vi "Get Index Directory Path.vi"(8 "error in (no error)":errorcluster) -> (0 "error out":errorcluster, 3 "Index Directory":path)   [LabVIEW 2020, in "Paths.lvlib"]
doc: "Generates the default configuration path. \nWhen called from the development environement, the default config path is the /Config relative to the project path.\nWhen called from a built exe the default config path is at C:\\Users\\<username>\\AppData\\Local\\<CompanyName>\\<ProductName> where company name and product name are the ones configured in the build specification.\nOn Linux the default config directory is \\home\\lvuser\\natinst\\bin\\config."
uses:
  Paths.lvlib
  <vilib>/Utility/sysdir.llb/System Directory Type.ctl
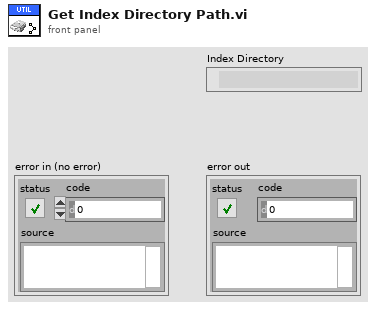
[diagram p1: front panel]
types:
  T1 = typedef "System Directory Type.ctl" = i32
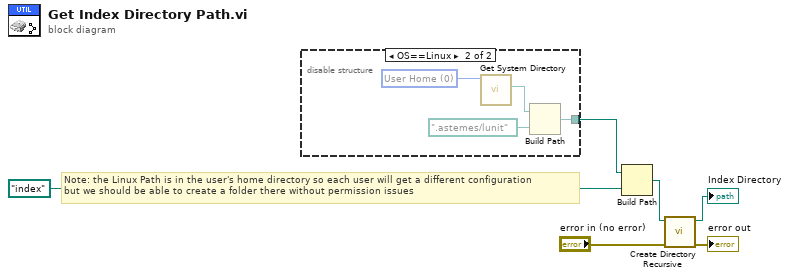
[diagram p0: block diagram]
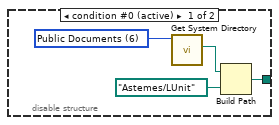
[diagram p2: hidden frame]
diagram:
  # "Note: the Linux Path is in the user's home directory so each user will get a different configuration \nbut we should be able to create a folder there without permission issues"
  n1 = disable-structure shown="OS==Linux" {
    disable-tunnel: [w10 w11] -> w3
    frame condition #0 (active) {
      w9 = T1 6 items=["User Home"=0, "User Desktop"=1, "User Documents"=2, "User Application Data"=3, "User Preferences"=4, "User Temporary"=5, "Public Documents"=6, "Public Application Data"=7, "Public Preferences"=8, "Public Cache"=13, "System Core Libraries"=9, "System Installed Libraries"=10, "Application Files"=11, "Boot Volume Root"=12] ("system directory type")
      n2 = call <vilib>:"Get System Directory.vi"("system directory type"=w9) -> ("system directory"=w7:path)  [unwired: 10 in]
      n3 = Build Path(base path=w7, name or relative path=path "Astemes/LUnit") -> (appended path=w10:path)
    }
    frame condition #1 {
      w14 = T1 0 items=["User Home"=0, "User Desktop"=1, "User Documents"=2, "User Application Data"=3, "User Preferences"=4, "User Temporary"=5, "Public Documents"=6, "Public Application Data"=7, "Public Preferences"=8, "Public Cache"=13, "System Core Libraries"=9, "System Installed Libraries"=10, "Application Files"=11, "Boot Volume Root"=12] ("system directory type")
      n4 = call <vilib>:"Get System Directory.vi"("system directory type"=w14) -> ("system directory"=w12:path)  [unwired: 10 in]
      n5 = Build Path(base path=w12, name or relative path=path ".astemes/lunit") -> (appended path=w11:path)
    }
  }
  n6 = Build Path(base path=w3, name or relative path=path "index") -> (appended path=w2:path)
  n7 = call <vilib>:"Create Directory Recursive.vi"("error in (no error)"="error in (no error)", "directory"=w2) -> ("error out"=→"error out":errorcluster, "directory copy"=→"Index Directory":path)  [unwired: 3 in, 1 out]
